vi "Find Command Names.vi"(11 "TargetItem in":refnum<vi>) -> (2 "Paths":path[](array[path]), 3 "Command Info":T2(array[cluster]))   [LabVIEW 2019]
uses:
  <vilib>/picture/picture.llb/imagedata.ctl
  <vilib>/Utility/Data Type/NI_Data Type.lvlib
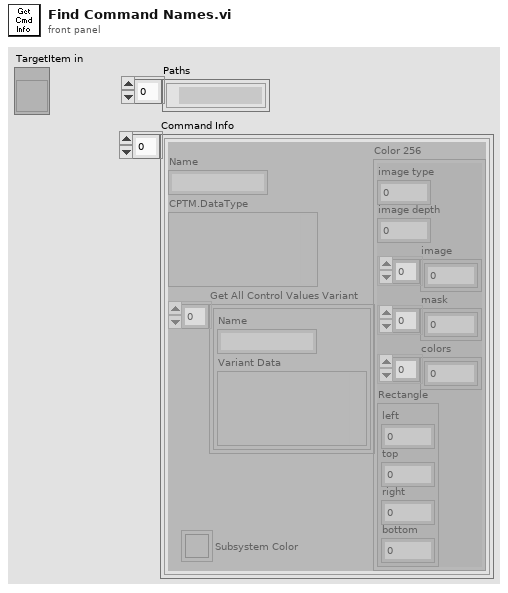
[diagram p1: front panel]
types:
  T1 = typedef "imagedata.ctl" = cluster{"image type":i32, "image depth":i32, "image":u8[], "mask":u8[], "colors":u32[], "Rectangle":cluster{"left":i16, "top":i16, "right":i16, "bottom":i16}}
  T2 = cluster{"Name":string, "CPTM.DataType":variant, "Get All Control Values Variant":cluster{"Name":string, "Variant Data":variant}[], "Color 256":T1, "Subsystem Color":u32}[]
  T3 = typedef "NI_Data Type.lvlib/Type Definition Info.ctl" = cluster{"Name":string, "Timestamp":u32}
  T4 = cluster{"Name":string, "CPTM.DataType":variant, "Get All Control Values Variant":cluster{"Name":string, "Variant Data":variant}[], "ImageData":T1, "Color Box":u32}
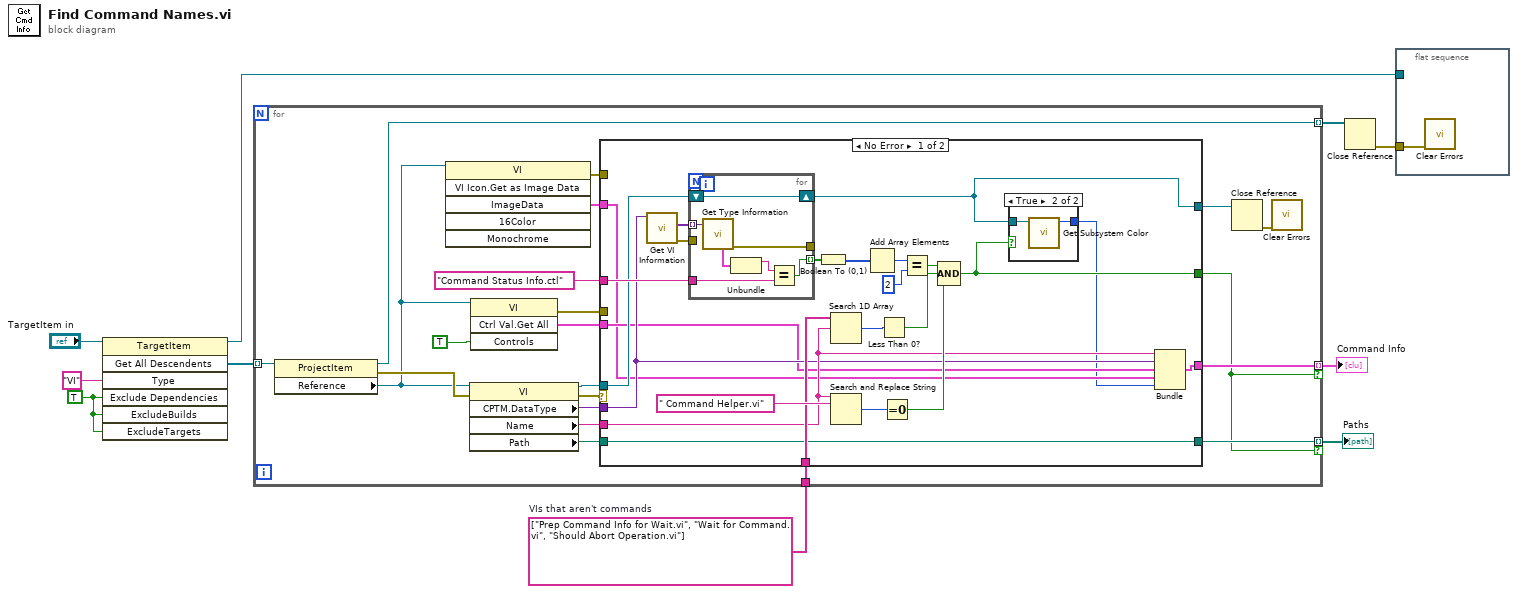
[diagram p0: block diagram]
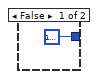
[diagram p2: hidden frame]
diagram:
  w7 = TRUE ("ExcludeDependencies")
  w5 = string[] ["Prep Command Info for Wait.vi", "Wait for Command.vi", "Should Abort Operation.vi"]  # VIs that aren't commands
  n1 = invoke class="TargetItem" method="Get All Descendents"(reference="TargetItem in", "Type"="VI", "Exclude Dependencies"=w7, "ExcludeBuilds"=w7, "ExcludeTargets"=w7) -> (reference out=w1:refnum<vi>, "All Descendents"=w8:refnum<vi>[])  [unwired: 2 in, 5 out]
  n2 = for {
    tunnel: w8 -> [w31] mode=indexing
    tunnel: w5 -> [w29]
    tunnel: [w22] -> w9 mode=indexing if=w19
    tunnel: [w20] -> w10 mode=indexing if=w19
    tunnel: [w12] -> w2 mode=indexing
    n3 = property class="ProjectItem"(reference=w31) -> (reference out=w12:refnum<vi>, error out=w24:errorcluster, "Reference"=w15:refnum<vi>)  [unwired: 1 in]
    n4 = invoke class="VI" method="VI Icon.Get as Image Data"(reference=w15) -> (error out=w13:errorcluster, "ImageData"=w14:T1)  [unwired: 5 in, 4 out]
    n5 = property class="VI"(reference=w15, error in=w24) -> (reference out=w11:refnum<vi>, error out=w23:errorcluster, "CPTM.DataType"=w28:variant, "Name"=w27:string, "Path"=w21:path)
    n6 = invoke class="VI" method="Ctrl Val.Get All"(reference=w15, "Controls"=TRUE) -> (error out=w16:errorcluster, "Get All Control Values Variant"=w17:cluster{"Name":string, "Variant Data":variant}[])  [unwired: 2 in, 2 out]
    n7 = case shown="No Error" w23 {
      tunnel: "Command Status Info.ctl" ("Name") -> [w44 _]
      tunnel: w29 -> [w43 _]
      tunnel: w28 -> [w37 _]
      tunnel: w27 -> [w39 _]
      tunnel: [w33 w66] -> w25
      tunnel: w11 -> [w41 w66]
      tunnel: [w38 _] -> w22
      tunnel: [w34 _] -> w19
      tunnel: w21 -> [w40 _]
      tunnel: [w40 _] -> w20
      tunnel: w17 -> [w36 _]
      tunnel: w16 -> [_ _]
      tunnel: w14 -> [w35 _]
      tunnel: w13 -> [_ _]
      frame No Error {
        n8 = call <vilib>:"Get VI Information.vi"("variant"=w37) -> ("error out"=w47:errorcluster, "VI terminal types"=w46:variant[])  [unwired: 7 in, 2 out]
        n9 = for {
          tunnel: w44 -> [w65]
          tunnel: [w64] -> w45 mode=indexing
          tunnel: w46 -> [w62] mode=indexing
          tunnel: w47 -> [_]
          tunnel: [w61] -> _
          shift-right: [w63] -> w33
          shift-left: w41 -> [w63]
          n10 = call <vilib>:"Get Type Information.vi"("variant"=w62) -> ("error out"=w61:errorcluster, "type definition info"=w60:T3)  [unwired: 6 in, 3 out]
          n11 = Unbundle(w60) -> ("Name"=w59:string)  [unwired: 1 out]
          n12 = Equal?(x=w59, y=w65) -> (x = y?=w64:bool)
        }
        n13 = Boolean To (0,1)(Boolean=w45) -> (0, 1=w42:i16[])
        n14 = Search 1D Array(1D array=w43, element=w39) -> (index of element=w50:i32)  [unwired: 1 in]
        n15 = Search and Replace String(input string=w39, search string=" Command Helper.vi") -> (number of replacements=w52:i32)  [unwired: 6 in, 3 out]
        n16 = Add Array Elements(numeric array=w42) -> (sum=w54:i16)
        n17 = Less Than 0?(x=w50) -> (x < 0?=w51:bool)
        n18 = Equal To 0?(x=w52) -> (x = 0?=w53:bool)
        n19 = Equal?(x=w54, y=2) -> (x = y?=w55:bool)
        n20 = Compound Arithmetic op=AND(w55, w51, w53) -> (w34:bool)
        n21 = case shown="True" w34 {
          tunnel: w33 -> [_ w58]
          tunnel: [u32 16777216 ("Color Box") w57] -> w32
          frame False {
          }
          frame True {
            n22 = call "Get Subsystem Color.vi"("VI in"=w58) -> ("Color Box"=w57:u32)  [unwired: 10 in]
          }
        }
        n23 = Bundle("Name"=w39, "CPTM.DataType"=w37, "Get All Control Values Variant"=w36, "ImageData"=w35, "Color Box"=w32) -> (w38:T4)  [unwired: 1 in]
      }
      frame Error {
      }
    }
    n24 = Close Reference(reference=w25) -> (error out=w26:errorcluster)  [unwired: 1 in]
    n25 = call <vilib>:"Clear Errors.vi"("error in (no error)"=w26) -> ()  [unwired: 5 in, 2 out]
  }
  "Paths" <- w10
  "Command Info" <- w9
  n26 = Close Reference(reference=w2) -> (error out=w3:errorcluster)  [unwired: 1 in]
  n27 = flat-sequence {
    tunnel: w3 -> [w67]
    tunnel: w1 -> [_]
    frame #0 {
      n28 = call <vilib>:"Clear Errors.vi"("error in (no error)"=w67) -> ()  [unwired: 5 in, 2 out]
    }
  }
